vi "set_duty_cycle.vi"(8 "error in (no error)":errorcluster, 10 "duty cycle":dbl[unit], 11 "DL090503StimulatorScaffold.lvclass in":refnum<class "StimulatorDL090503Scaffold.lvclass">) -> (0 "error out":errorcluster, 3 "DL090503StimulatorScaffold.lvclass out":refnum<class "StimulatorDL090503Scaffold.lvclass">)   [LabVIEW 2010, in "StimulatorDL090503Scaffold.lvclass"]
uses:
  StimulatorDL090503Scaffold.lvclass
  StimulatorDL090503Scaffold.lvclass/StimulatorDL090503Scaffold.ctl
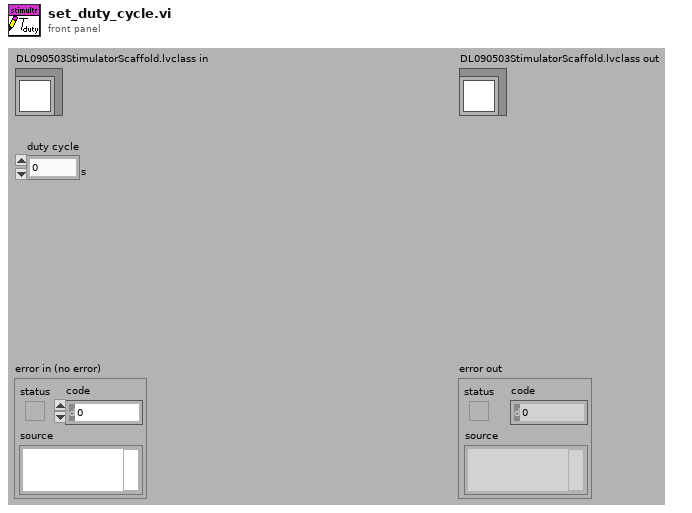
[diagram p1: front panel]
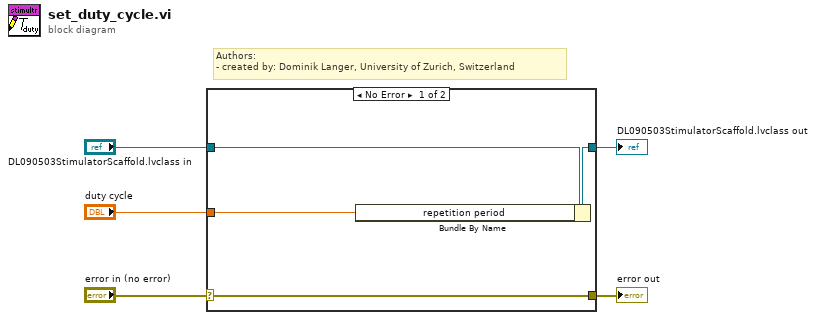
[diagram p0: block diagram]
diagram:
  # "Authors: \n- created by: Dominik Langer, University of Zurich, Switzerland"
  n1 = case shown="No Error" "error in (no error)" {
    selector: "error in (no error)" -> [w9 w10]
    tunnel: [w9 w10] -> w4
    tunnel: [w7 w11] -> w2
    tunnel: "DL090503StimulatorScaffold.lvclass in" -> [w8 w11]
    tunnel: "duty cycle" -> [w6 _]
    frame No Error {
      n2 = Bundle By Name(cluster=w8, "repetition period"=w6) -> (w7:refnum<class "StimulatorDL090503Scaffold.lvclass">)
    }
    frame Error {
    }
  }
  "error out" <- w4
  "DL090503StimulatorScaffold.lvclass out" <- w2
